vi "Reset.vi"(8 "error in (no error)":errorcluster, 10 "Message in":refnum<class "ResetMessage.lvclass">, 11 "BMC in":refnum<class "BMC.lvclass">) -> (0 "error out":errorcluster, 3 "BMC out":refnum<class "BMC.lvclass">)   [LabVIEW 2012, in "BMC.lvclass"]
doc: "The reset method processes the command 'reset'. \n\nResets the internal state of the component (without performing a full initialisation). This could be resetting hardware, or private data to default values."
uses:
  BMC.lvclass
  <vilib>/Distrio/Murmex/ResetMessage/ResetMessage.lvclass
  <vilib>/Distrio/Murmex/Murmex/Murmex.lvclass
  BMC.lvclass/BMC.ctl
panel:
  # "This method is called when the RESET\ntrigger is sent. \n\nOverride this method when your component needs to\nrespond to this trigger. \n\nCall parent for proper implementation"
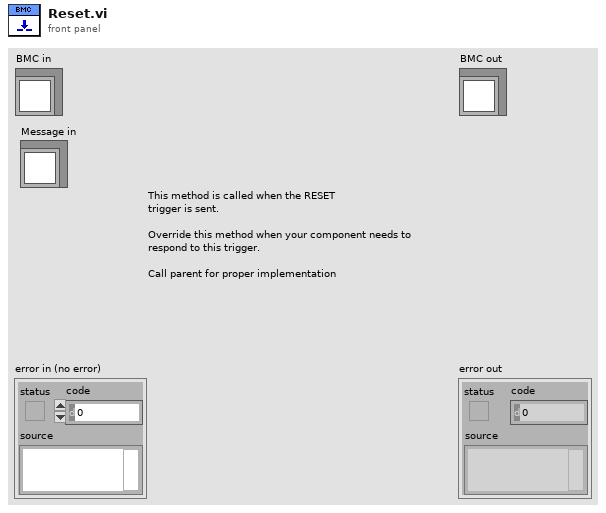
[diagram p1: front panel]
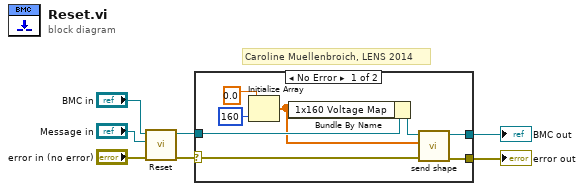
[diagram p0: block diagram]
diagram:
  # "Caroline Muellenbroich, LENS 2014"
  n1 = call-parent "Reset.vi"("error in (no error)"="error in (no error)", "Message in"="Message in", "Murmex in"="BMC in") -> ("error out"=w4:errorcluster, "Murmex out"=w2:refnum<class "BMC.lvclass">)  [unwired: 7 in]
  n2 = case shown="No Error" w4 {
    selector: w4 -> [w13 w16]
    tunnel: [w15 w16] -> w3
    tunnel: w2 -> [w12 w17]
    tunnel: [w14 w17] -> w1
    frame No Error {
      n3 = Initialize Array(0.0 ("element"), 160 ("dimension size")) -> (w8:dbl[])
      n4 = Bundle By Name(cluster=w12, "1x160 Voltage Map"=w8) -> (w11:refnum<class "BMC.lvclass">)
      n5 = call-dynamic "send shape.vi"("error in (no error)"=w13, "1x160 Voltage Map"=w8, "BMC in"=w11) -> ("error out"=w15:errorcluster, "BMC out"=w14:refnum<class "BMC.lvclass">)  [unwired: 7 in]
    }
    frame Error {
    }
  }
  "error out" <- w3
  "BMC out" <- w1
